vi "Temperature Controller.vi"(8 "error in (no error)":errorcluster, 11 "Temperature Controller in":refnum<class "Temperature Controller.lvclass">) -> (0 "error out":errorcluster, 3 "Temperature Controller out":refnum<class "Temperature Controller.lvclass">)   [LabVIEW 2017, in "Temperature Controller.lvclass"]
uses:
  Temperature Controller.lvclass
  C:/LabVIEW-programs-dev/Instruments/Utility Classes/Readable/Readable.lvclass
  Utility Classes/Readable/Channel Units.ctl
  Temperature Controller.lvclass/Temperature Controller.ctl
  Global/GPIB Numbers.vi
  Utility Classes/Readable/Readable.lvclass
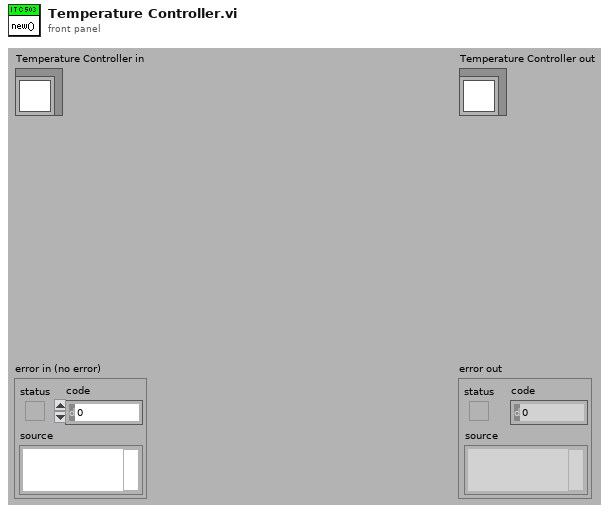
[diagram p1: front panel]
types:
  T1 = typedef "ITCIO.ctl" = cluster{"Address":T2, "Version":T3, "Ch 1 dec places":i16, "Ch 2 dec places":i16, "Ch 3 dec places":i16, "Ch1 Name":string, "Ch2 Name":string, "Ch3 Name":string}
  T2 = typedef "OxfordAddress.ctl" = cluster{"Com Port":i32, "ISOBUS Address":i32, "GPIB Address":i16, "Communication":enum16{"RS232", "ISOBUS", "GPIB", "Gateway"}}
  T3 = typedef "ITCVersion.ctl" = enum16{"ITC502", "ITC503", "ITC601"}
  T4 = typedef "Readable.lvclass/Channel Units.ctl" = string[]
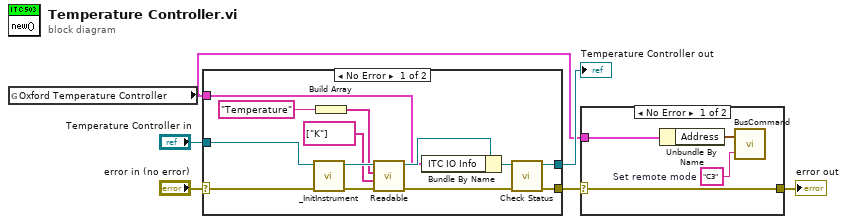
[diagram p0: block diagram]
diagram:
  n1 = global read "GPIB Numbers.vi" "Oxford Temperature Controller"() -> (w3:T1)
  n2 = case shown="No Error" "error in (no error)" {
    selector: "error in (no error)" -> [w14 w21]
    tunnel: [w16 w21] -> w2
    tunnel: [w17 w20] -> w4
    tunnel: "Temperature Controller in" -> [w19 w20]
    tunnel: w3 -> [w7 _]
    frame No Error {
      n3 = call-dynamic "_InitInstrument.vi"("error in (no error)"=w14, "Instrument in"=w19) -> ("error out"=w12:errorcluster, "Instrument out"=w15:refnum<class "Temperature Controller.lvclass">)  [unwired: 8 in]
      n4 = Build Array("Temperature") -> (w8:string[])
      n5 = call "Readable.vi"("error in (no error)"=w12, "Channel Units"=T4 ["K"], "Channel Names"=w8, "Readable in"=w15) -> ("error out"=w11:errorcluster, "Readable out"=w13:refnum<class "Temperature Controller.lvclass">)  [unwired: 6 in]
      n6 = Bundle By Name(cluster=w13, "ITC IO Info"=w7) -> (w18:refnum<class "Temperature Controller.lvclass">)
      n7 = call-dynamic "Check Status.vi"("error in (no error)"=w11, "Temperature Controller in"=w18) -> ("error out"=w16:errorcluster, "Temperature Controller out"=w17:refnum<class "Temperature Controller.lvclass">)  [unwired: 6 in, 2 out]
    }
    frame Error {
    }
  }
  "Temperature Controller out" <- w4
  n8 = case shown="No Error" w2 {
    selector: w2 -> [w25 w26]
    tunnel: [w25 w26] -> w1
    tunnel: w3 -> [w22 _]
    frame No Error {
      w24 = "C3"  # Set remote mode
      n9 = Unbundle By Name(w22) -> ("Address"=w23:T2)
      n10 = call "BusCommand.vi"("Command"=w24, "Instrument address (in)"=w23) -> ()  [unwired: 2 out]
    }
    frame Error {
    }
  }
  "error out" <- w1
